vi "Tree.AddProperties.vi"(7 "Report Passed?":bool, 8 "error in (no error)":errorcluster, 9 "Parent":string, 10 "Properties":variant, 11 "Tree Ref":refnum<vi>) -> (0 "error out":errorcluster, 2 "Passed?":bool, 3 "Tree Ref":refnum<vi>)   [LabVIEW 2015, in "Analysis.lvlib"]
uses:
  Analysis.lvlib
  Types/Analysis.PropertyGroups.ctl
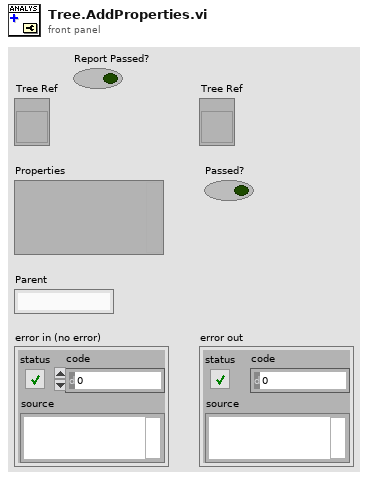
[diagram p1: front panel]
types:
  T1 = typedef "Analysis.lvlib/Analysis.PropertyGroups.ctl" = cluster{"Pass":bool, "Additional Info":variant}
  T2 = typedef "Type Descriptor Enumeration__ogtk.ctl" = enum8{"<Null>", "I8", "I16", "I32", "I64", "U8", "U16", "U32", "U64", "SGL", "DBL", "EXT", "CSG", "CDB", "CXT", "0x0F", "0x10", "0x11", "0x12", "0x13", "0x14", "Enum U8", "Enum U16", "Enum U32", "Enum U64", "SGL PQ", "DBL PQ", "EXT PQ", "CSG PQ", "CDB PQ", "CXT PQ", "0x1F", "0x20", "Boolean", "0x22", "0x23", "0x24", "0x25", "0x26", "0x27", "0x28", "0x29", "0x2A", "0x2B", "0x2C", "0x2D", "0x2E", "0x2F", "String", "0x31", "Path", "Pict", "0x34", "0x35", "0x36", "DAQ", "0x38", "0x39", "0x3A", "0x3B", "0x3C", "0x3D", "0x3E", "0x3F", "Array", "0x41", "0x42", "0x43", "0x44", "0x45", "0x46", "0x47", "0x48", "0x49", "0x4A", "0x4B", "0x4C", "0x4D", "0x4E", "0x4F", "Cluster", "0x51", "0x52", "Variant", "Waveform", "0x55", "0x56", "0x57", "0x58", "0x59", "0x5A", "0x5B", "0x5C", "0x5D", "0x5E", "0x5F", "0x60", "0x61", "0x62", "0x63", "0x64", "0x65", "0x66", "0x67", "0x68", "0x69", "0x6A", "0x6B", "0x6C", "0x6D", "0x6E", "0x6F", "Refnum"}
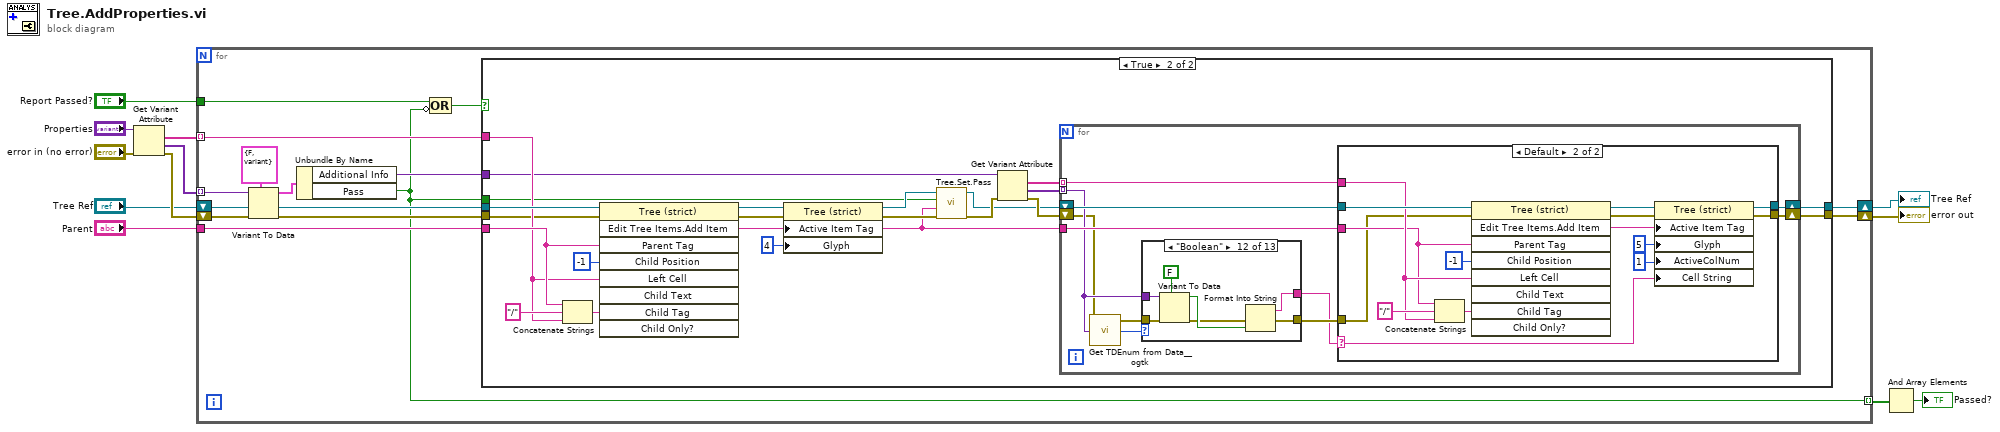
[diagram p0: block diagram]
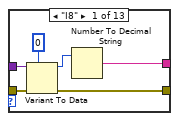
[diagram p4: hidden frame]
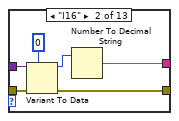
[diagram p5: hidden frame]
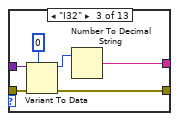
[diagram p6: hidden frame]
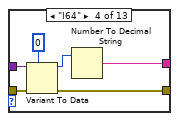
[diagram p7: hidden frame]
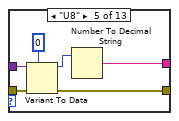
[diagram p8: hidden frame]
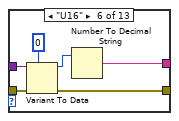
[diagram p9: hidden frame]
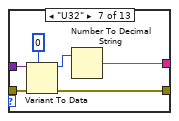
[diagram p10: hidden frame]
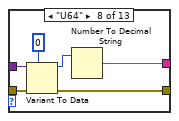
[diagram p11: hidden frame]
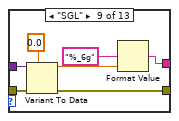
[diagram p12: hidden frame]
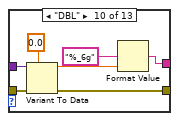
[diagram p13: hidden frame]
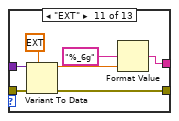
[diagram p14: hidden frame]
diagram:
  n1 = Get Variant Attribute(Variant="Properties", error in="error in (no error)") -> (names=w11:string[], values=w10:variant[], error out=w9:errorcluster)  [unwired: 2 in, 1 out]
  n2 = for {
    tunnel: "Parent" -> [w25]
    shift-right: [w16] -> w2
    shift-left: w9 -> [w20]
    shift-right: [w17] -> w3
    shift-left: "Tree Ref" -> [w26]
    tunnel: [w14] -> w4 mode=indexing
    tunnel: w10 -> [w22] mode=indexing
    tunnel: w11 -> [w23] mode=indexing
    tunnel: "Report Passed?" -> [w15]
    n3 = Variant To Data(error in=w20, type=T1 {"Pass"=FALSE, "Additional Info"=variant}, Variant=w22) -> (data=w21:T1, error out=w19:errorcluster)
    n4 = Unbundle By Name(w21) -> ("Additional Info"=w18:variant, "Pass"=w14:bool)
    n5 = Compound Arithmetic op=OR(w15, invert w14) -> (w13:bool)
    n6 = case shown="True" w13 {
      tunnel: w26 -> [w27 w49]
      tunnel: w25 -> [_ w47]
      tunnel: w23 -> [_ w40]
      tunnel: w19 -> [w28 w38]
      tunnel: w18 -> [_ w37]
      tunnel: [w27 w32] -> w17
      tunnel: [w28 w31] -> w16
      tunnel: w14 -> [_ w29]
      frame False {
      }
      frame True {
        n7 = Concatenate Strings(w47, "/" ("string"), w40) -> (w46:string)
        n8 = invoke class="Tree (strict)" method="Edit Tree Items.Add Item"(reference=w49, error in=w38, "Parent Tag"=w47, "Child Position"=-1, "Left Cell"=w40, "Child Tag"=w46) -> (reference out=w43:refnum<vi>, error out=w44:errorcluster, "Edit Tree Items:Add Item"=w33:string)  [unwired: 3 in, 6 out]
        n9 = property class="Tree (strict)"(reference=w43, error in=w44, "Active Item Tag"=w33, "Glyph"=4 ("Active Item:Symbol Index")) -> (reference out=w42:refnum<vi>, error out=w39:errorcluster)
        n10 = call "Tree.Set.Pass.vi"("error in (no error)"=w39, "Edit Tree Items:Add Item"=w33, "Passed"=w29, "TreeControl in"=w42) -> ("error out"=w36:errorcluster, "TreeControl out"=w32:refnum<vi>)  [unwired: 6 in]
        n11 = Get Variant Attribute(Variant=w37, error in=w36) -> (names=w35:string[], values=w30:variant[], error out=w34:errorcluster)  [unwired: 2 in, 1 out]
        n12 = for {
          tunnel: w35 -> [w59] mode=indexing
          tunnel: w33 -> [w58]
          shift-right: [w56] -> _
          shift-left: w32 -> [w57]
          shift-right: [w55] -> w31
          shift-left: w34 -> [w52]
          tunnel: w30 -> [w53] mode=indexing
          n13 = call <userlib>:"Get TDEnum from Data__ogtk.vi"("Data"=w53) -> ("Type Descriptor Enumeration"=w54:T2)  [unwired: 4 in]
          n14 = case shown="\"Boolean\"" w54 {
            tunnel: w53 -> [w82 w88 w94 w100 w106 w112 w118 w124 w131 w138 w145 w152 _]
            tunnel: w52 -> [w79 w85 w91 w97 w103 w109 w115 w121 w129 w136 w143 w150 w153]
            tunnel: [w78 w84 w90 w96 w102 w108 w114 w120 w125 w132 w139 w148 _] -> w50
            tunnel: [w77 w83 w89 w95 w101 w107 w113 w119 w128 w135 w142 w146 w153] -> w51
            frame "I8" {
              n15 = Variant To Data(error in=w79, type=i8 0 ("default (0 I32)"), Variant=w82) -> (data=w80:i8, error out=w77:errorcluster)
              n16 = Number To Decimal String(number=w80) -> (decimal integer string=w78:string)  [unwired: 1 in]
            }
            frame "I16" {
              n17 = Variant To Data(error in=w85, type=i16 0 ("default (0 I32)"), Variant=w88) -> (data=w86:i16, error out=w83:errorcluster)
              n18 = Number To Decimal String(number=w86) -> (decimal integer string=w84:string)  [unwired: 1 in]
            }
            frame "I32" {
              n19 = Variant To Data(error in=w91, type=0 ("default (0 I32)"), Variant=w94) -> (data=w92:i32, error out=w89:errorcluster)
              n20 = Number To Decimal String(number=w92) -> (decimal integer string=w90:string)  [unwired: 1 in]
            }
            frame "I64" {
              n21 = Variant To Data(error in=w97, type=i64 0 ("default (0 I32)"), Variant=w100) -> (data=w98:i64, error out=w95:errorcluster)
              n22 = Number To Decimal String(number=w98) -> (decimal integer string=w96:string)  [unwired: 1 in]
            }
            frame "U8" {
              n23 = Variant To Data(error in=w103, type=u8 0 ("default (0 I32)"), Variant=w106) -> (data=w104:u8, error out=w101:errorcluster)
              n24 = Number To Decimal String(number=w104) -> (decimal integer string=w102:string)  [unwired: 1 in]
            }
            frame "U16" {
              n25 = Variant To Data(error in=w109, type=u16 0 ("default (0 I32)"), Variant=w112) -> (data=w110:u16, error out=w107:errorcluster)
              n26 = Number To Decimal String(number=w110) -> (decimal integer string=w108:string)  [unwired: 1 in]
            }
            frame "U32" {
              n27 = Variant To Data(error in=w115, type=u32 0 ("default (0 I32)"), Variant=w118) -> (data=w116:u32, error out=w113:errorcluster)
              n28 = Number To Decimal String(number=w116) -> (decimal integer string=w114:string)  [unwired: 1 in]
            }
            frame "U64" {
              n29 = Variant To Data(error in=w121, type=u64 0 ("default (0 I32)"), Variant=w124) -> (data=w122:u64, error out=w119:errorcluster)
              n30 = Number To Decimal String(number=w122) -> (decimal integer string=w120:string)  [unwired: 1 in]
            }
            frame "SGL" {
              n31 = Variant To Data(error in=w129, type=sgl 0.0 ("default (0 I32)"), Variant=w131) -> (data=w126:sgl, error out=w128:errorcluster)
              n32 = Format Value(format string="%_6g", value (0)=w126) -> (output string=w125:string)  [unwired: 1 in]
            }
            frame "DBL" {
              n33 = Variant To Data(error in=w136, type=0.0 ("default (0 I32)"), Variant=w138) -> (data=w133:dbl, error out=w135:errorcluster)
              n34 = Format Value(format string="%_6g", value (0)=w133) -> (output string=w132:string)  [unwired: 1 in]
            }
            frame "EXT" {
              n35 = Variant To Data(error in=w143, type=ext 0.0 ("default (0 I32)"), Variant=w145) -> (data=w140:ext, error out=w142:errorcluster)
              n36 = Format Value(format string="%_6g", value (0)=w140) -> (output string=w139:string)  [unwired: 1 in]
            }
            frame "Boolean" {
              n37 = Variant To Data(error in=w150, type=FALSE, Variant=w152) -> (data=w149:bool, error out=w147:errorcluster)
              n38 = Format Into String(error in=w147, w149) -> (resulting string=w148:string, error out=w146:errorcluster)  [unwired: 2 in]
            }
            frame Default {
            }
          }
          n39 = case shown="Default" w50 {
            selector: w50 -> [_ w62]
            tunnel: w59 -> [_ w71]
            tunnel: w58 -> [_ w70]
            tunnel: w57 -> [w60 w67]
            tunnel: [w60 w66] -> w56
            tunnel: [w61 w65] -> w55
            tunnel: w51 -> [w61 w63]
            frame "" {
            }
            frame Default {
              n40 = Concatenate Strings(w70, "/" ("string"), w71) -> (w73:string)
              n41 = invoke class="Tree (strict)" method="Edit Tree Items.Add Item"(reference=w67, error in=w63, "Parent Tag"=w70, "Child Position"=-1, "Left Cell"=w71, "Child Tag"=w73) -> (reference out=w68:refnum<vi>, error out=w69:errorcluster, "Edit Tree Items:Add Item"=w75:string)  [unwired: 3 in, 6 out]
              n42 = property class="Tree (strict)"(reference=w68, error in=w69, "Active Item Tag"=w75, "Glyph"=5 ("Active Item:Symbol Index"), "ActiveColNum"=1 ("Active Cell:Active Column Number"), "Cell String"=w62) -> (reference out=w66:refnum<vi>, error out=w65:errorcluster)
            }
          }
        }
      }
    }
  }
  "Tree Ref" <- w3
  "error out" <- w2
  n43 = And Array Elements(Boolean array=w4) -> (logical AND=→"Passed?":bool)
